vi "SetParam.vi"(8 "error in (no error)":errorcluster caption="entrée d'erreur (pas d'erreur)", 10 "precision_recall_curve":T1={"pos_label"={"dtype_pos_label"="None", "pos_label"="None"}, "sample_weight"=[], "Returns"="precision"}, 11 "Precision_Recall_Curve.lvclass":refnum<class "Precision_Recall_Curve.lvclass">) -> (0 "error out":errorcluster caption="sortie d'erreur", 3 "Precision_Recall_Curve.lvclass":refnum<class "Precision_Recall_Curve.lvclass">)   [LabVIEW 2020, in "Precision_Recall_Curve.lvclass"]
doc: "Set Parameters"
uses:
  Precision_Recall_Curve.lvclass
  Precision_Recall_Curve.lvclass/Precision_Recall_Curve.ctl
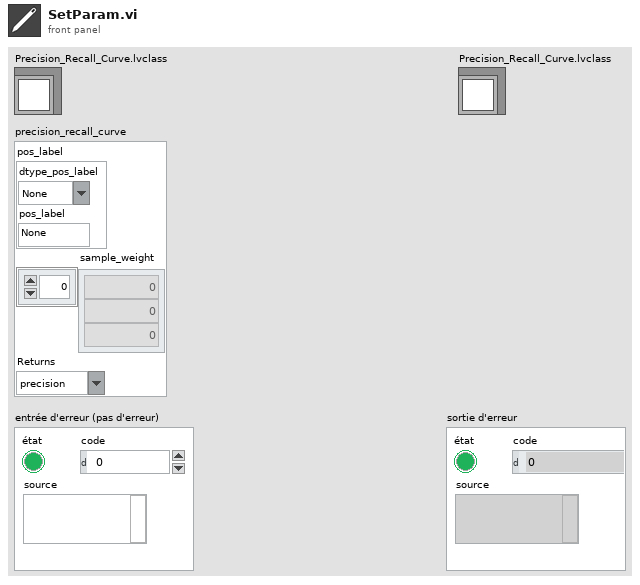
[diagram p1: front panel]
types:
  T1 = cluster{"pos_label":cluster{"dtype_pos_label":string, "pos_label":string}, "sample_weight":dbl[], "Returns":string}
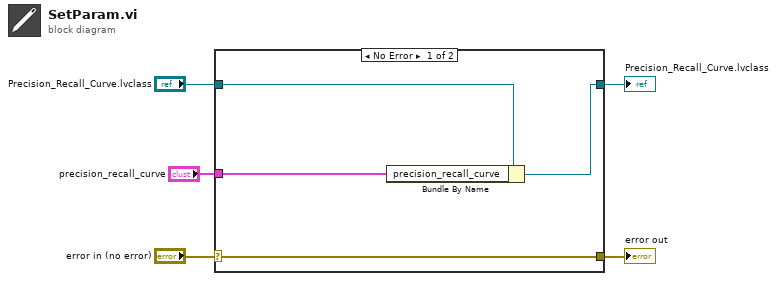
[diagram p0: block diagram]
diagram:
  n1 = case shown="No Error" "error in (no error)" {
    selector: "error in (no error)" -> [w9 w10]
    tunnel: [w9 w10] -> w4
    tunnel: [w7 w11] -> w2
    tunnel: "Precision_Recall_Curve.lvclass" -> [w8 w11]
    tunnel: "precision_recall_curve" -> [w6 _]
    frame No Error {
      n2 = Bundle By Name(cluster=w8, "precision_recall_curve"=w6) -> (w7:refnum<class "Precision_Recall_Curve.lvclass">)
    }
    frame Error {
    }
  }
  "error out" <- w4
  "Precision_Recall_Curve.lvclass" <- w2
